vi "Write using Data Attributes.vi"() -> ()   [LabVIEW 2022 SP3]
uses:
  <vilib>/express/express shared/transition.llb/Dynamic To Waveform Array.vi
  <vilib>/express/express signal manip/GetorSetDDTAttributes/Set DDT Attributes/SetT0.vi
  <vilib>/express/express shared/transition.llb/Waveform Array To Dynamic.vi
  <vilib>/express/express signal manip/GetorSetDDTAttributes/Set DDT Attributes/Set DDT Properties.xnode
panel:
  in  "Write to Excel":bool
  in  "Frequency":dbl
  in  "Power":dbl
  in  "Current":dbl
  in  "Voltage":dbl
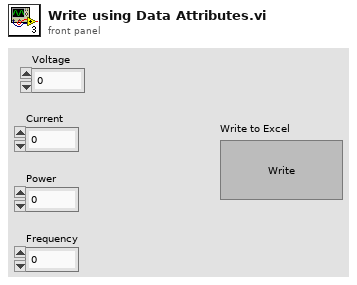
[diagram p1: front panel]
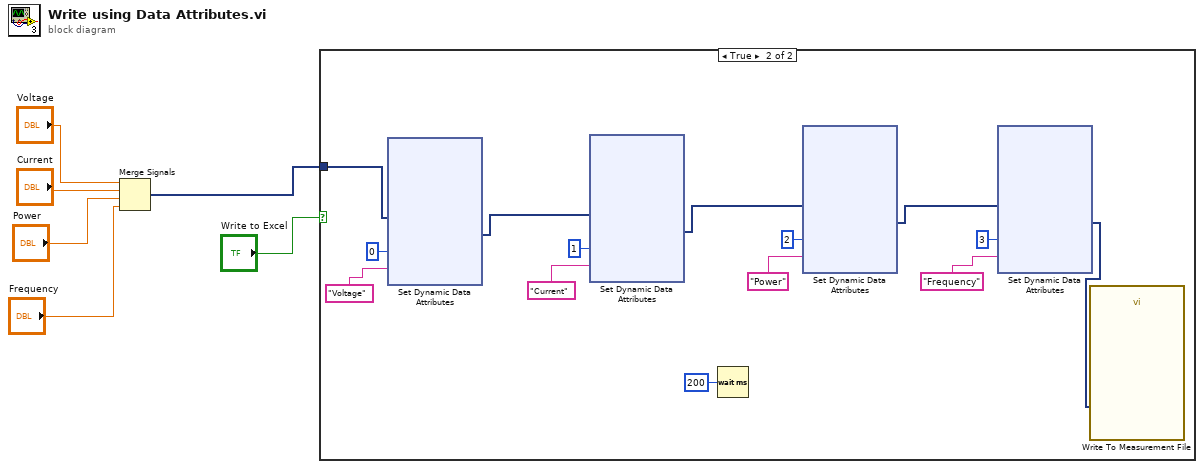
[diagram p0: block diagram]
diagram:
  n1 = Merge Signals("Voltage", "Current", "Power", "Frequency") -> (w1:dynamicdata)
  n2 = case shown="True" "Write to Excel" {
    tunnel: w1 -> [_ w11]
    frame False {
    }
    frame True {
      n3 = xnode "Set Dynamic Data Attributes"("Signals In"=w11, "Signal Index"=0, "Signal Name"="Voltage") -> ("Signals Out"=w10:dynamicdata)  [unwired: 1 in, 1 out]
      n4 = xnode "Set Dynamic Data Attributes"("Signals In"=w10, "Signal Index"=1, "Signal Name"="Current") -> ("Signals Out"=w9:dynamicdata)  [unwired: 1 in, 1 out]
      n5 = Wait (ms)(milliseconds to wait=u32 200) -> ()  [unwired: 1 out]
      n6 = xnode "Set Dynamic Data Attributes"("Signals In"=w9, "Signal Index"=2, "Signal Name"="Power") -> ("Signals Out"=w8:dynamicdata)  [unwired: 1 in, 1 out]
      n7 = xnode "Set Dynamic Data Attributes"("Signals In"=w8, "Signal Index"=3, "Signal Name"="Frequency") -> ("Signals Out"=w7:dynamicdata)  [unwired: 1 in, 1 out]
      n8 = call "Write To Measurement File"("Signals"=w7) -> ()  [unwired: 16 in, 3 out]
    }
  }
